vi "Timer_GetTimer_t0.vi"() -> (16 "Timer.t0":u16)   [LabVIEW 2018]
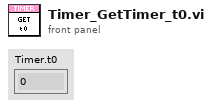
[diagram p1: front panel]
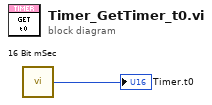
[diagram p0: block diagram]
diagram:
  n1 = call "16 Bit mSec"() -> ("Tick Count(mSec)"=→"Timer.t0":u16)
